vi "SubVI_Angulos_motores.vi"(1 "input cluster":T1) -> (0 "output cluster":T1)   [LabVIEW 2017]
panel:
  out "Ângulo":dbl
  out "Angulo 2":dbl
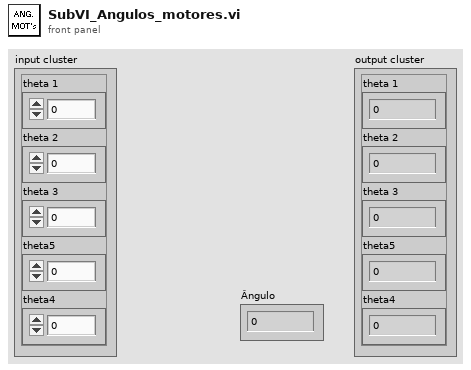
[diagram p1: front panel]
types:
  T1 = cluster{"theta 1":dbl, "theta 2":dbl, "theta 3":dbl, "theta5":dbl, "theta4":dbl}
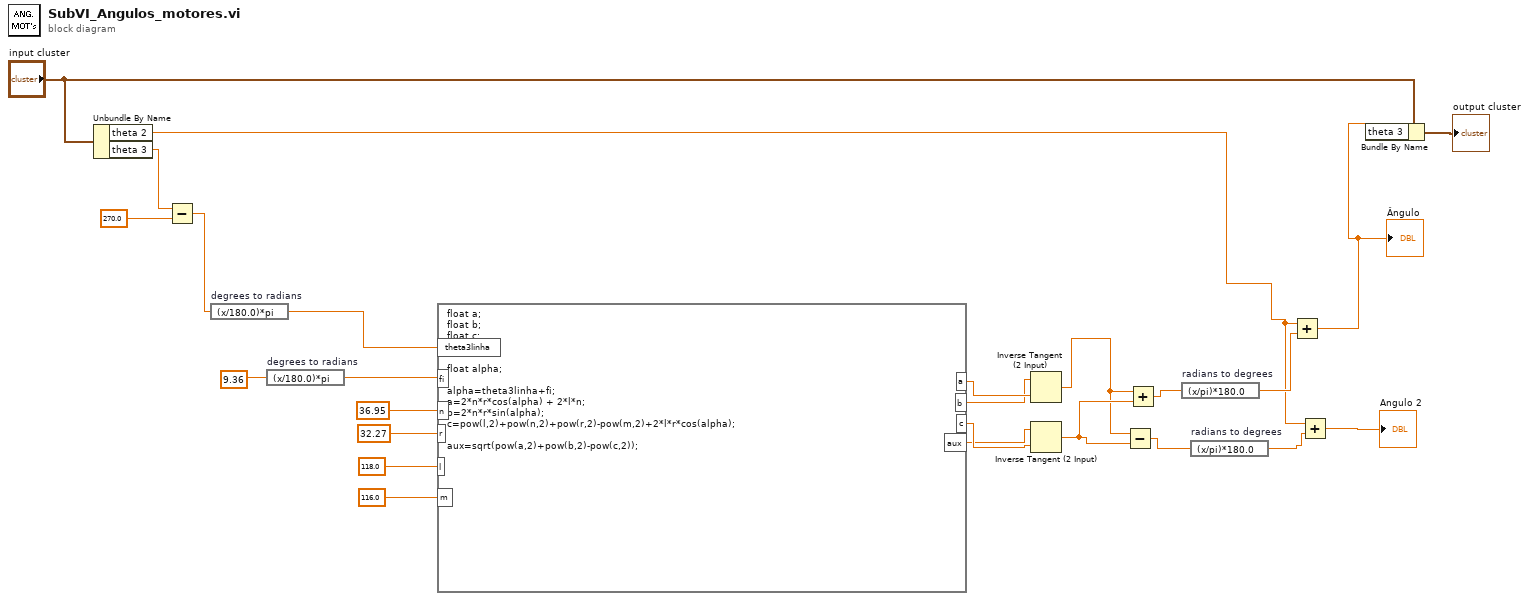
[diagram p0: block diagram]
diagram:
  n1 = Unbundle By Name("input cluster") -> ("theta 2"=w4:dbl, "theta 3"=w5:dbl)
  n2 = Subtract(x=w5, y=270.0) -> (x-y=w10:dbl)
  n3 = expression code="(x/180.0)*pi" "degrees to radians"(w10) -> (w17:dbl)
  n4 = expression code="(x/180.0)*pi" "degrees to radians"(9.36 ("input variable")) -> (w19:dbl)
  n5 = formula code="float a;\nfloat b;\nfloat c;\nfloat aux;\n\nfloat alpha;\n\nalpha=theta3linha+fi;\na=2*n*r*cos(alpha) + 2*l*n;\nb=2*n*r*sin(alpha);\nc=pow(l,2)+pow(n,2)+pow(r,2)-pow(m,2)+2*l*r*cos(alpha);\n\naux=sqrt(pow(a,2)+pow(b,2)-pow(c,2));"("theta3linha"=w17, "fi"=w19, "n"=36.95 ("input variable"), "r"=32.27 ("input variable"), "l"=118.0 ("input variable"), "m"=116.0 ("input variable")) -> ("a"=w16:dbl, "b"=w15:dbl, "c"=w21:dbl, "aux"=w20:dbl)
  n6 = Inverse Tangent (2 Input)(1:w16, 2:w15) -> (0:w22:dbl)
  n7 = Inverse Tangent (2 Input)(1:w21, 2:w20) -> (0:w23:dbl)
  n8 = Subtract(x=w22, y=w23) -> (x-y=w25:dbl)
  n9 = Add(x=w22, y=w23) -> (x+y=w24:dbl)
  n10 = expression code="(x/pi)*180.0" "radians to degrees"(w24) -> (w8:dbl)
  n11 = expression code="(x/pi)*180.0" "radians to degrees"(w25) -> (w7:dbl)
  n12 = Add(x=w4, y=w8) -> (x+y=w3:dbl)
  "Ângulo" <- w3
  n13 = Add(x=w4, y=w7) -> (x+y=→"Angulo 2":dbl)
  n14 = Bundle By Name(cluster="input cluster", "theta 3"=w3) -> (→"output cluster":T1)
